vi "Estimate All Positions - Swarm Method.vi"(0 "TagArray In":refnum<class "Tag.lvclass">[](array[class]), 1 "AllTagDistancesArray":T2(array[cluster]), 2 "AltTDA":T2(array[cluster]), 3 "Werkpunten":T5(array[cluster]), 5 "AnchorsArray":refnum<class "Anchor.lvclass">[](array[class]), 7 "error in (no error)":errorcluster) -> (13 "error out":errorcluster, 15 "Solution Vector":dbl[](array[numeric]) format="%.2f", 17 "SwarmOutputArray":T4(array[cluster]))   [LabVIEW 2014]
uses:
  Tag.lvclass
  Anchor/Anchor.lvclass
  <vilib>/Analysis/Matrix/Datatypes/RealMatrix.ctl
  <vilib>/Analysis/baseanly.llb/Matrix Type of Inverse Matrix.ctl
  <vilib>/Analysis/7linalg.llb/Solve Linear Equations (single right hand).vi
  <vilib>/Analysis/baseanly.llb/Solve Linear Equations By Cholesky.vi
  <vilib>/Analysis/baseanly.llb/Real Matrix to Compact Array.vi
  <vilib>/Analysis/baseanly.llb/Real Compact Tri-Matrix Linear Eqs.vi
  <vilib>/Analysis/Matrix/Numeric/Conversions/Array To Matrix - RA2.vi
  <vilib>/Analysis/7linalg.llb/Solve Linear Eqs (General).vi
  <vilib>/Analysis/7linalg.llb/Solve Linear Eqs (Gen, single right hand).vi
  <vilib>/Analysis/NI_AALPro.lvlib
  <vilib>/Analysis/NI_AALBase.lvlib
  <vilib>/Analysis/Matrix/NI_Matrix.lvlib
panel:
  out "fSwarmOutputArray":T1(array[cluster])
  out "RealSolutionVector":dbl[](array[numeric])
  out "Solution Vector AnchorToTag":dbl[](array[numeric]) format="%.2f"
  out "Solution Vector TagToTag":dbl[](array[numeric]) format="%.2f"
  out "Known Vector 3":T3
  out "Known Vector 2":T3
  out "Known Vector 1":T3
  out "Input Matrix 2":T3
  out "Input Matrix 1":T3
  out "Results Real":T3
  out "Input Matrix 3":T3
  out "# tags":i32=22
  out "Tag To":i32
  out "TagIDFrom":dbl format="%.2f"
  # "Output Indicators"
  # "Input Controls"
  # "Error Control"
  # "Error Indicator"
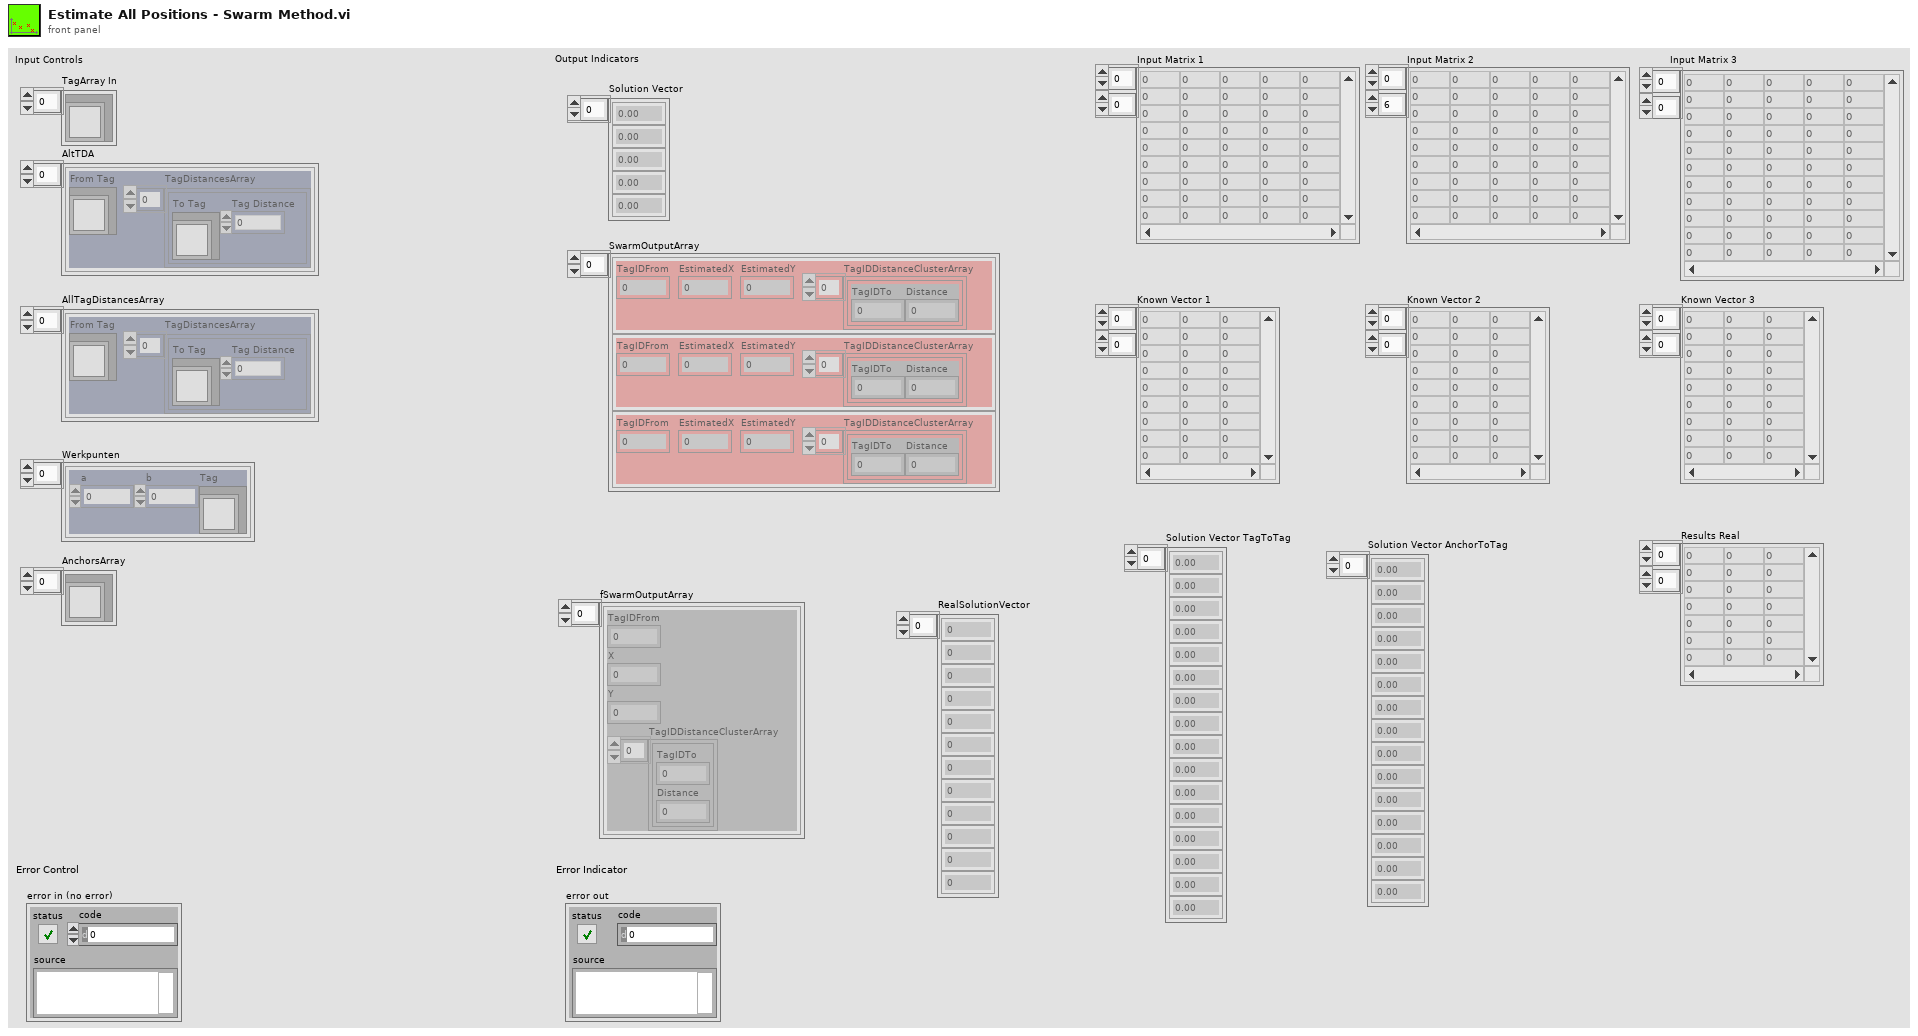
[diagram p1: front panel]
types:
  T1 = cluster{"TagIDFrom":dbl, "X":dbl, "Y":dbl, "TagIDDistanceClusterArray":cluster{"TagIDTo":dbl, "Distance":dbl}[]}[]
  T2 = cluster{"From Tag":refnum<class "Tag.lvclass">, "TagDistancesArray":cluster{"To Tag":refnum<class "Tag.lvclass">, "Tag Distance":dbl}[]}[]
  T3 = typedef "NI_Matrix.lvlib/RealMatrix.ctl" = dbl[][]
  T4 = cluster{"TagIDFrom":dbl, "EstimatedX":dbl, "EstimatedY":dbl, "TagIDDistanceClusterArray":cluster{"TagIDTo":dbl, "Distance":dbl}[]}[]
  T5 = cluster{"a":dbl, "b":dbl, "Tag":refnum<class "Tag.lvclass">}[]
  T6 = typedef "NI_AALBase.lvlib/Matrix Type of Inverse Matrix.ctl" = enum32{"General", "Positive Definite", "Lower Triangular", "Upper Triangular"}
  T7 = cluster{"Tag.lvclass":refnum<class "Tag.lvclass">, "Distance":dbl}[]
  T8 = cluster{"a":dbl, "b":dbl, "Tag":refnum<class "Tag.lvclass">}
  T9 = cluster{"From Tag":refnum<class "Tag.lvclass">, "TagDistancesArray":cluster{"To Tag":refnum<class "Tag.lvclass">, "Tag Distance":dbl}[]}
  T10 = cluster{"To Tag":refnum<class "Tag.lvclass">, "Tag Distance":dbl}[]
  T11 = cluster{"To Tag":refnum<class "Tag.lvclass">, "Tag Distance":dbl}
  T12 = cluster{"TagID":dbl, dbl, dbl, "TagIDDistanceClusterArray":cluster{"TagIDTo":dbl, "Distance":dbl}[]}
  T13 = cluster{"TagID":dbl, "X":dbl, "Y":dbl, "TagIDDistanceClusterArray":cluster{"TagIDTo":dbl, "Distance":dbl}[]}[]
  T14 = cluster{"TagIDFrom":dbl, "X":dbl, "Y":dbl, "TagIDDistanceClusterArray":cluster{"TagIDTo":dbl, "Distance":dbl}[]}
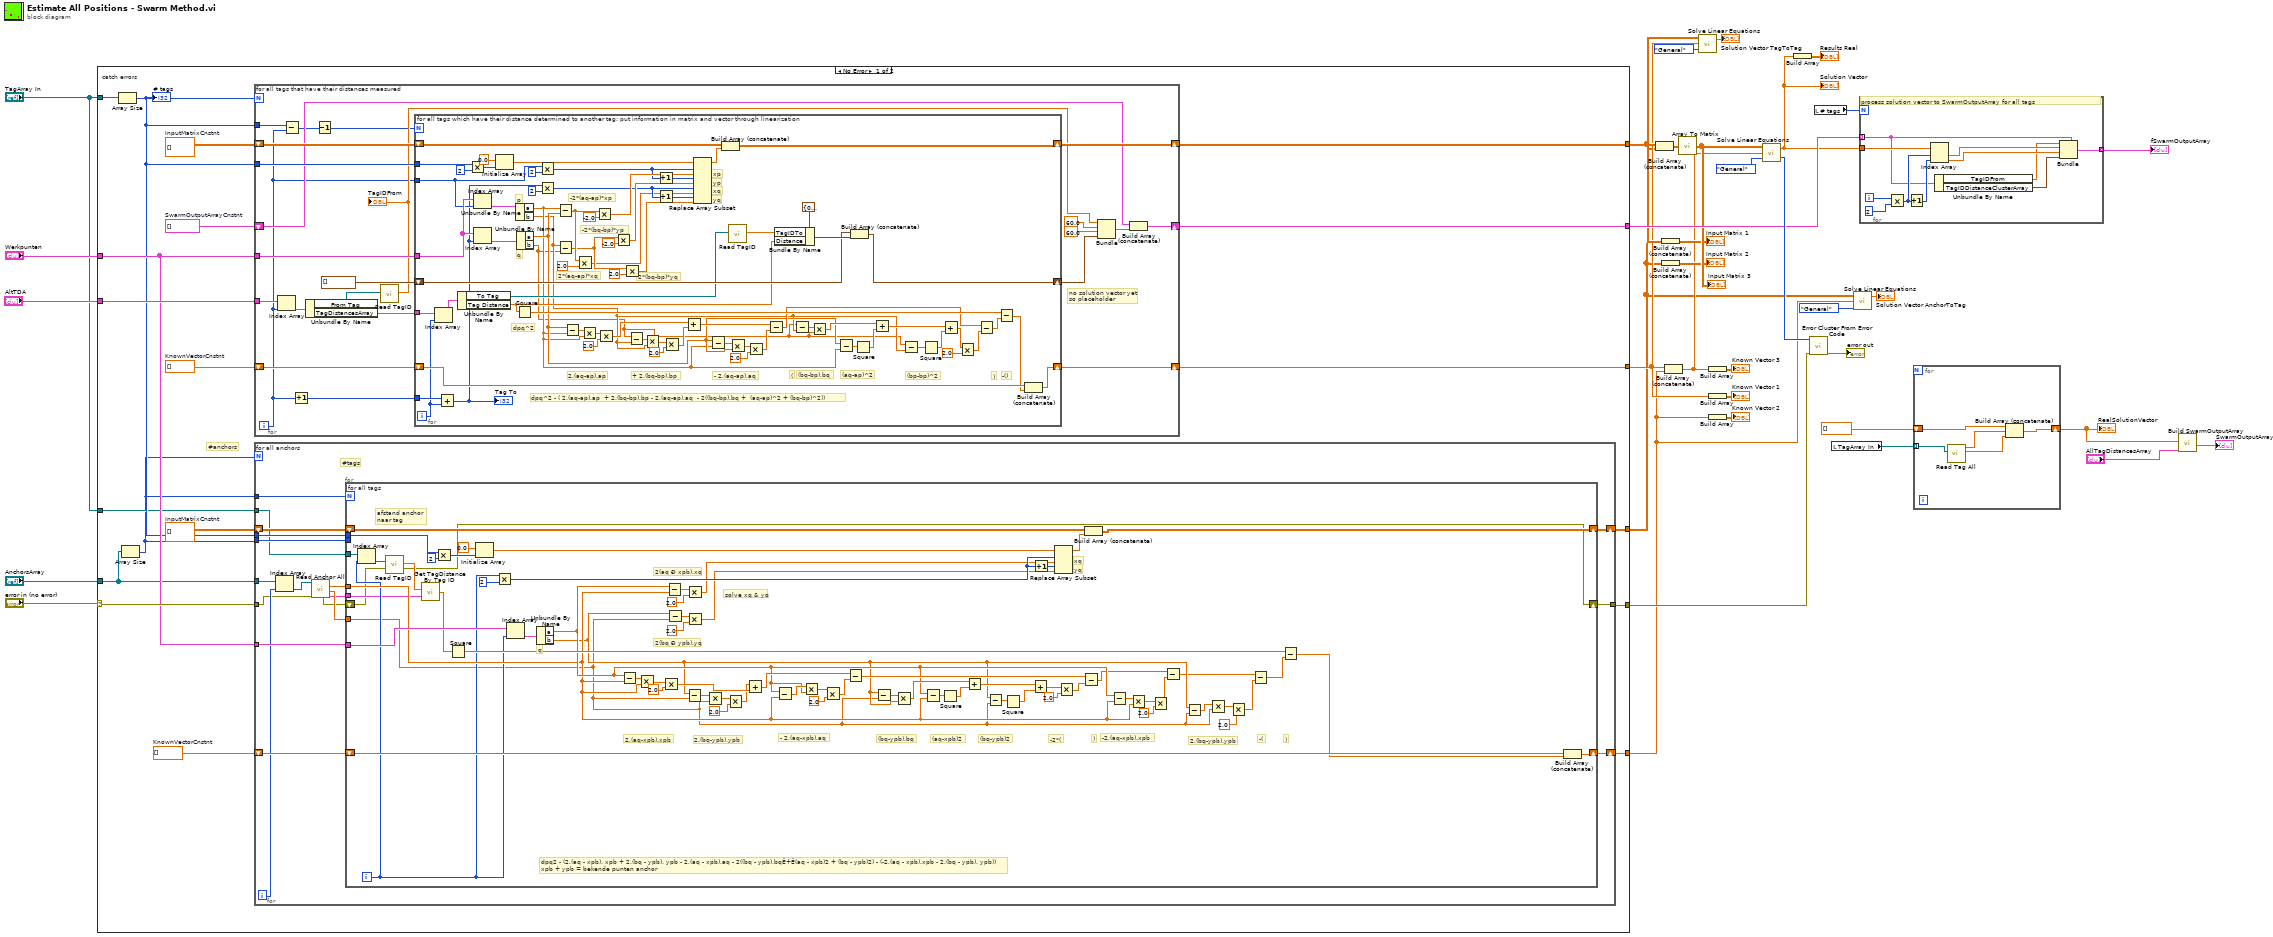
[diagram p0: block diagram]
diagram:
  n1 = case shown="No Error" "error in (no error)" {
    selector: "error in (no error)" -> [w48 w239]
    tunnel: [w53 _] -> w13
    tunnel: "Werkpunten" -> [w40 _]
    tunnel: "AnchorsArray" -> [w38 _]
    tunnel: [w51 _] -> w14
    tunnel: [w50 _] -> w9
    tunnel: [w49 _] -> w8
    tunnel: "TagArray In" -> [w43 _]
    tunnel: [w47 w239] -> w30
    tunnel: [w45 _] -> w28
    tunnel: "AltTDA" -> [w44 _]
    tunnel: "TagArray In" -> [w37 _]
    frame No Error {
      w41 = dbl[] []  # KnownVectorCnstnt
      w42 = dbl[][] []  # InputMatrixCnstnt
      w46 = T1 []  # SwarmOutputArrayCnstnt
      w52 = dbl[] []  # KnownVectorCnstnt
      w54 = dbl[][] []  # InputMatrixCnstnt
      # "#anchors"
      # "catch errors"
      n2 = Array Size(array=w43) -> (size(s)=w39:i32)
      "# tags" <- w39
      n3 = Array Size(array=w38) -> (size(s)=w36:i32)
      n4 = for {
        N: w36 -> [_]
        tunnel: w39 -> [w71]
        tunnel: w40 -> [w72]
        tunnel: w39 -> [w70]
        tunnel: w36 -> [w69]
        tunnel: w38 -> [w61]
        shift-right: [w68] -> w50
        shift-left: w42 -> [w67]
        shift-right: [w65] -> w49
        shift-left: w41 -> [w66]
        tunnel: w48 -> [w58]
        tunnel: [w64] -> w47
        tunnel: w37 -> [w56]
        i -> [w62]
        # "#tags"
        # "for all anchors"
        n5 = Index Array(array=w61, index=w62) -> (element=w63:refnum<class "Anchor.lvclass">)
        n6 = call "Read Anchor All.vi"("error in (no error)"=w58, "Anchor in"=w63) -> ("TagDistanceArray"=w55:T7, "AnchorY"=w60:dbl, "AnchorX"=w59:dbl, "error out"=w57:errorcluster)  [unwired: 4 in, 2 out]
        n7 = for {
          N: w71 -> [_]
          tunnel: w72 -> [w142]
          tunnel: w69 -> [_]
          tunnel: w70 -> [w137]
          shift-right: [w141] -> w68
          shift-left: w67 -> [w140]
          shift-right: [w139] -> w65
          shift-left: w66 -> [w138]
          shift-right: [w81] -> w64
          shift-left: w57 -> [w82]
          tunnel: w60 -> [w76]
          tunnel: w59 -> [w94]
          tunnel: w56 -> [w86]
          tunnel: w55 -> [w83]
          i -> [w84]
          # "afstand anchor \nnaar tag"
          # "2.(bq-ypb).ypb"
          # "-2.(aq-xpb).xpb"
          # ")"
          # "-("
          # "(bq-ypb)2"
          # "(aq-xpb)2"
          # "(bq-ypb).bq"
          # ")"
          # "-2*("
          # "- 2.(aq-xpb).aq"
          # "2.(bq-ypb).ypb"
          # "2.(aq-xpb).xpb"
          # "solve xq & yq"
          # "2(bq Ð ypb).yq"
          # "2(aq Ð xpb).xq"
          # "dpq2 - (2.(aq - xpb). xpb + 2.(bq - ypb). ypb - 2.(aq - xpb).aq - 2((bq - ypb).bqÊ+Ê(aq - xpb)2 + (bq - ypb)2) - (-2.(aq - xpb).xpb - 2.(bq - ypb). ypb))\nxpb + ypb = bekende punten anchor"
          # "yq"
          # "xq"
          # "q"
          # "for all tags"
          n8 = Index Array(array=w86, index=w84) -> (element=w85:refnum<class "Tag.lvclass">)
          n9 = call "Read TagID.vi"("Tag in"=w85, "error in (no error)"=w82) -> ("TagID"=w88:dbl, "error out"=w81:errorcluster)  [unwired: 15 in, 1 out]
          n10 = call "Get TagDistance By Tag ID.vi"("TagID"=w88, "TagDistanceArray"=w83) -> ("Distance"=w87:dbl)  [unwired: 13 in]
          n11 = Multiply(x=w137, y=2) -> (x*y=w129:i32)
          n12 = Square(x=w87) -> (x^2=w121:dbl)
          n13 = Initialize Array(0.0 ("element"), w129) -> (w133:dbl[])
          n14 = Multiply(x=w84, y=2) -> (x*y=w128:i32)
          n15 = Index Array(array=w142, index=w84) -> (element=w132:T8)
          n16 = Unbundle By Name(w132) -> ("a"=w96:dbl, "b"=w91:dbl)
          n17 = Subtract(x=w96, y=w94) -> (x-y=w120:dbl)
          n18 = Multiply(x=w120, y=w94) -> (x*y=w119:dbl)
          n19 = Multiply(x=w119, y=2.0) -> (x*y=w117:dbl)
          n20 = Subtract(x=w96, y=w94) -> (x-y=w127:dbl)
          n21 = Subtract(x=w91, y=w76) -> (x-y=w124:dbl)
          n22 = Subtract(x=w91, y=w76) -> (x-y=w116:dbl)
          n23 = Multiply(x=w127, y=2.0) -> (x*y=w125:dbl)
          n24 = Multiply(x=w124, y=2.0) -> (x*y=w122:dbl)
          n25 = Multiply(x=w116, y=w76) -> (x*y=w115:dbl)
          n26 = Multiply(x=w115, y=2.0) -> (x*y=w113:dbl)
          n27 = Add(x=w113, y=w117) -> (x+y=w112:dbl)
          n28 = Subtract(x=w96, y=w94) -> (x-y=w111:dbl)
          n29 = Multiply(x=w111, y=w96) -> (x*y=w110:dbl)
          n30 = Multiply(x=w110, y=2.0) -> (x*y=w108:dbl)
          n31 = Subtract(x=w112, y=w108) -> (x-y=w107:dbl)
          n32 = Subtract(x=w91, y=w76) -> (x-y=w104:dbl)
          n33 = Multiply(x=w104, y=w91) -> (x*y=w103:dbl)
          n34 = Subtract(x=w96, y=w94) -> (x-y=w101:dbl)
          n35 = Square(x=w101) -> (x^2=w102:dbl)
          n36 = Add(x=w103, y=w102) -> (x+y=w98:dbl)
          n37 = Subtract(x=w91, y=w76) -> (x-y=w100:dbl)
          n38 = Square(x=w100) -> (x^2=w99:dbl)
          n39 = Add(x=w98, y=w99) -> (x+y=w97:dbl)
          n40 = Increment(x=w128) -> (x+1=w130:i32)
          n41 = Replace Array Subset(array=w133, new element #1=w125, index #1=w128, new element #2=w122, index #2=w130) -> (w134:dbl[])
          n42 = Multiply(x=w97, y=2.0) -> (x*y=w105:dbl)
          n43 = Subtract(x=w107, y=w105) -> (x-y=w79:dbl)
          n44 = Build Array (concatenate)(w140, w134) -> (w141:dbl[][])
          n45 = Subtract(x=w96, y=w94) -> (x-y=w95:dbl)
          n46 = Multiply(x=w95, y=w94) -> (x*y=w93:dbl)
          n47 = Multiply(x=w93, y=2.0) -> (x*y=w80:dbl)
          n48 = Subtract(x=w79, y=w80) -> (x-y=w74:dbl)
          n49 = Subtract(x=w91, y=w76) -> (x-y=w90:dbl)
          n50 = Multiply(x=w90, y=w76) -> (x*y=w77:dbl)
          n51 = Multiply(x=w77, y=2.0) -> (x*y=w75:dbl)
          n52 = Subtract(x=w74, y=w75) -> (x-y=w73:dbl)
          n53 = Subtract(x=w121, y=w73) -> (x-y=w89:dbl)
          n54 = Build Array (concatenate)(w138, w89) -> (w139:dbl[])
        }
      }
      n55 = for {
        N: w39 -> [_]
        tunnel: w39 -> [w165]
        shift-right: [w162] -> w51
        shift-left: w54 -> [w163]
        tunnel: w39 -> [w161]
        tunnel: w40 -> [w160]
        shift-right: [w159] -> w53
        shift-left: w52 -> [w158]
        shift-right: [w153] -> w45
        shift-left: w46 -> [w154]
        tunnel: w44 -> [w147]
        i -> [w145]
        # "no solution vector yet\nso placeholder"
        # "for all tags that have their distances measured"
        n56 = Index Array "Index Array"(array=w147, index=w145) -> (element=w146:T9)
        n57 = Subtract(x=w165, y=w145) -> (x-y=w148:i32)
        n58 = Increment(x=w145) -> (x+1=w164:i32)
        n59 = Unbundle By Name(w146) -> ("From Tag"=w144:refnum<class "Tag.lvclass">, "TagDistancesArray"=w150:T10)
        n60 = Decrement(x=w148) -> (x-1=w143:i32)
        n61 = call "Read TagID.vi"("Tag in"=w144) -> ("TagID"=w149:dbl)  [unwired: 16 in, 2 out]
        "TagIDFrom" <- w149
        n62 = for {
          N: w143 -> [_]
          tunnel: w164 -> [w238]
          shift-right: [w237] -> w162
          shift-left: w163 -> [w231]
          tunnel: w161 -> [w233]
          tunnel: w160 -> [w177]
          tunnel: w145 -> [w176]
          shift-right: [w210] -> w159
          shift-left: w158 -> [w211]
          shift-right: [w179] -> w155
          shift-left: cluster{"TagIDTo":dbl, "Distance":dbl}[] [] ("TagIDDistanceClusterArray") -> [w180]
          tunnel: w150 -> [w172]
          i -> [w171]
          # ")"
          # "("
          # "2*(bq-bp)*yq"
          # "2*(aq-ap)*xq"
          # "-2*(bq-bp)*yp"
          # "-2*(aq-ap)*xp"
          # "yq"
          # "xq"
          # "yp"
          # "xp"
          # "(bp-bp)^2"
          # "(aq-ap)^2"
          # "-()"
          # "p"
          # "q"
          # "dpq^2"
          # "(bq-bp).bq"
          # "- 2.(aq-ap).aq"
          # "+ 2.(bq-bp).bp"
          # "2.(aq-ap).ap"
          # "dpq^2 - ( 2.(aq-ap).ap  + 2.(bq-bp).bp - 2.(aq-ap).aq  - 2((bq-bp).bq +  (aq-ap)^2 + (bq-bp)^2))"
          # "for all tags which have their distance determined to another tag: put information in matrix and vector through linearization"
          n63 = Index Array(array=w172, index=w171) -> (element=w170:T11)
          n64 = Add(x=w238, y=w171) -> (x+y=w173:i32)
          "Tag To" <- w173
          n65 = Unbundle By Name(w170) -> ("To Tag"=w174:refnum<class "Tag.lvclass">, "Tag Distance"=w178:dbl)
          n66 = Multiply(x=w233, y=2) -> (x*y=w236:i32)
          n67 = Index Array "Index Array"(array=w177, index=w176) -> (element=w229:T8)
          n68 = Index Array "Index Array"(array=w177, index=w173) -> (element=w228:T8)
          n69 = Initialize Array "Initialize Array"(0.0 ("element"), w236) -> (w230:dbl[])
          n70 = Unbundle By Name(w229) -> ("a"=w168:dbl, "b"=w167:dbl)
          n71 = Square(x=w178) -> (x^2=w209:dbl)
          n72 = Unbundle By Name(w228) -> ("a"=w169:dbl, "b"=w166:dbl)
          n73 = Multiply(x=w176, y=2) -> (x*y=w222:i32)
          n74 = Multiply(x=w173, y=2) -> (x*y=w219:i32)
          n75 = Subtract(x=w168, y=w169) -> (x-y=w215:dbl)
          n76 = Subtract(x=w167, y=w166) -> (x-y=w214:dbl)
          n77 = Subtract(x=w169, y=w168) -> (x-y=w207:dbl)
          n78 = Multiply(x=w215, y=2.0) -> (x*y=w213:dbl)
          n79 = Multiply(x=w207, y=w168) -> (x*y=w206:dbl)
          n80 = Multiply(x=w215, y=-2.0) -> (x*y=w225:dbl)
          n81 = Multiply(x=w206, y=2.0) -> (x*y=w205:dbl)
          n82 = Multiply(x=w214, y=-2.0) -> (x*y=w223:dbl)
          n83 = Multiply(x=w214, y=2.0) -> (x*y=w212:dbl)
          n84 = Subtract(x=w166, y=w167) -> (x-y=w204:dbl)
          n85 = Multiply(x=w204, y=w167) -> (x*y=w203:dbl)
          n86 = Increment(x=w222) -> (x+1=w221:i32)
          n87 = Increment(x=w219) -> (x+1=w218:i32)
          n88 = Multiply(x=w203, y=2.0) -> (x*y=w201:dbl)
          n89 = Add(x=w205, y=w201) -> (x+y=w197:dbl)
          n90 = Replace Array Subset(array=w230, new element #1=w225, index #1=w222, new element #2=w223, index #2=w221, new element #3=w213, index #3=w219, new element #4=w212, index #4=w218) -> (w232:dbl[])
          n91 = Subtract(x=w169, y=w168) -> (x-y=w200:dbl)
          n92 = Build Array (concatenate)(w231, w232) -> (w237:dbl[][])
          n93 = call "Read TagID.vi"("Tag in"=w174) -> ("TagID"=w175:dbl)  [unwired: 16 in, 2 out]
          n94 = Multiply(x=w200, y=w169) -> (x*y=w199:dbl)
          n95 = Multiply(x=w199, y=2.0) -> (x*y=w196:dbl)
          n96 = Subtract(x=w197, y=w196) -> (x-y=w184:dbl)
          n97 = Bundle By Name(cluster=cluster{"TagIDTo":dbl, "Distance":dbl} {"TagIDTo"=0.0, "Distance"=0.0} ("TagIDDistanceCluster"), "TagIDTo"=w175, "Distance"=w178) -> (w181:cluster{"TagIDTo":dbl, "Distance":dbl})
          n98 = Subtract(x=w166, y=w167) -> (x-y=w192:dbl)
          n99 = Multiply(x=w192, y=w166) -> (x*y=w191:dbl)
          n100 = Subtract(x=w169, y=w168) -> (x-y=w190:dbl)
          n101 = Build Array (concatenate)(w180, w181) -> (w179:cluster{"TagIDTo":dbl, "Distance":dbl}[])
          n102 = Square(x=w190) -> (x^2=w189:dbl)
          n103 = Add(x=w191, y=w189) -> (x+y=w188:dbl)
          n104 = Subtract(x=w166, y=w167) -> (x-y=w187:dbl)
          n105 = Square(x=w187) -> (x^2=w186:dbl)
          n106 = Add(x=w188, y=w186) -> (x+y=w185:dbl)
          n107 = Multiply(x=w185, y=2.0) -> (x*y=w194:dbl)
          n108 = Subtract(x=w184, y=w194) -> (x-y=w183:dbl)
          n109 = Subtract(x=w209, y=w183) -> (x-y=w195:dbl)
          n110 = Build Array (concatenate)(w211, w195) -> (w210:dbl[])
        }
        n111 = Bundle("TagID"=w149, 60.0, 60.0, "TagIDDistanceClusterArray"=w155) -> (w152:T12)  [unwired: 1 in]
        n112 = Build Array (concatenate)(w154, w152) -> (w153:T13)
      }
    }
    frame Error {
    }
  }
  n113 = Build Array (concatenate)(w14, w9) -> (w24:dbl[][])
  n114 = Build Array (concatenate)(w14) -> (→"Input Matrix 1":T3)
  n115 = Build Array (concatenate)(w9) -> (→"Input Matrix 2":T3)
  n116 = Build Array (concatenate)(w13, w8) -> (w16:dbl[])
  n117 = call-poly <vilib>:"Array To Matrix.vi"("Real 2D Array"=w24) -> ("Real Matrix"=w23:T3)
  "Input Matrix 3" <- w23
  n118 = call-poly <vilib>:"Solve Linear Equations.vi"("matrix type"=Matrix_Type_of_Inverse_Matrix."General", "Known Vector"=w13, "Input Matrix"=w14) -> ("Solution Vector"=→"Solution Vector TagToTag":dbl[])  [unwired: 1 out]
  n119 = Build Array(w16) -> (→"Known Vector 3":T3)
  n120 = Build Array(w13) -> (→"Known Vector 1":T3)
  n121 = Build Array(w8) -> (→"Known Vector 2":T3)
  n122 = call-poly <vilib>:"Solve Linear Equations.vi"("matrix type"=Matrix_Type_of_Inverse_Matrix."General", "Known Vector"=w16, "Input Matrix"=w23) -> ("error"=w31:i32, "Solution Vector"=w22:dbl[])
  "Solution Vector" <- w22
  n123 = Build Array(w22) -> (→"Results Real":T3)
  n124 = call <vilib>:"Error Cluster From Error Code.vi"("error in (no error)"=w30, "error code (0)"=w31) -> ("error out"=→"error out":errorcluster)  [unwired: 7 in]
  n125 = local read "# tags"() -> (w27:i32)
  n126 = local read "TagArray In"() -> (w5:refnum<class "Tag.lvclass">[])
  n127 = call-poly <vilib>:"Solve Linear Equations.vi"("matrix type"=Matrix_Type_of_Inverse_Matrix."General", "Known Vector"=w8, "Input Matrix"=w9) -> ("Solution Vector"=→"Solution Vector AnchorToTag":dbl[])  [unwired: 1 out]
  n128 = for {
    N: w27 -> [_]
    tunnel: w28 -> [w242] mode=indexing
    tunnel: [w243] -> w1 mode=indexing
    tunnel: w22 -> [w250]
    i -> [w249]
    # "process solution vector to SwarmOutputArray for all tags"
    n129 = Multiply(x=w249, y=2) -> (x*y=w247:i32)
    n130 = Increment(x=w247) -> (x+1=w246:i32)
    n131 = Index Array(array=w250, index #1=w247, index #2=w246) -> (element #1=w245:dbl, element #2=w244:dbl)
    n132 = Unbundle By Name(w242) -> ("TagIDFrom"=w241:dbl, "TagIDDistanceClusterArray"=w240:cluster{"TagIDTo":dbl, "Distance":dbl}[])
    n133 = Bundle(cluster=w242, "TagIDFrom"=w241, "X"=w245, "Y"=w244, "TagIDDistanceClusterArray"=w240) -> (w243:T14)
  }
  "fSwarmOutputArray" <- w1
  n134 = for {
    shift-right: [w254] -> w4
    shift-left: dbl[] [] ("RealSolutionVector") -> [w255]
    tunnel: w5 -> [w253] mode=indexing
    n135 = call "Read Tag All.vi"("Tag.lvclass"=w253) -> ("TagY"=w251:dbl, "TagX"=w252:dbl)  [unwired: 5 in, 4 out]
    n136 = Build Array (concatenate)(w255, w252, w251) -> (w254:dbl[])
  }
  "RealSolutionVector" <- w4
  n137 = call "Build SwarmOutputArray.vi"("AllTagDistancesArray"="AllTagDistancesArray", "Solution Vector"=w4) -> ("SwarmOutputArray"=→"SwarmOutputArray":T4)  [unwired: 9 in]
